vi "TURCK GUI TestPanel alle Module.vi"() -> ()   [LabVIEW 2017]
doc: "Example for reading and writing values for the TBEN-S2-2RFID-4DXP module from Turck"
uses:
  KH TURCK ETHERNETIP TDef Enum RFID Error.ctl
  KH TURCK ETHERNETIP TDefCluster TBEN-S2-2RFID-4DXP Status.ctl
  KH EthernetIPConfig 17.14/KH EthernetIPConfig TDef Config.ctl
  KH EthernetIPConfig 17.14/KH EthernetIPConfig TypeDefs ModuleTyp.ctl
  KH_DAQ 17.04/Turck/KH_DAQ_TURCK_TypeDefs_Cluster DI.ctl
  KH_DAQ 17.04/KH_DAQ_TypeDefs_Cluster AO.ctl
  KH_DAQ 17.04/KH_DAQ_TypeDefs_Messbereich.ctl
  KH_DAQ 17.04/KH_DAQ_TypeDefs_Bereich.ctl
  KH_DAQ 17.04/KH_DAQ_TypeDefs_Cluster AI.ctl
  KH TURCK ETHERNETIP TDef Enum IOL Data.ctl
  KH_DAQ 17.04/Turck/KH_DAQ_TURCK_TypeDefs_Cluster DO.ctl
  KH TURCK ETHERNETIP TDef Enum RFID Data RFID.ctl
  KH TURCK TypeDefs FGlob.ctl
  KH TURCK ETHERNETIP TDef Enum RFID User Command.ctl
  KH EthernetIP 17.19/KH_EthernetIP_Globals.vi
  KH TURCK ETHERNETIP RFID Global.vi
  KH TURCK ETHERNETIP RFID ST READ Global.vi
  KH TURCK ETHERNETIP Global.vi
panel:
  in  "Tab Control":T1(tab)
  in  "EIP_DO":T2={"Def"=[], "Signal Name"=["IOL1", "IOL3", "ARFID2", "ARFID3", "BRFID0", "BRFID1", "ADXP0", "ADXP2", "ADXP6", "ADXP7", "BDXP1", "BDXP2", "BDXP3", "BDXP7"], "Description"=[], "Chan"=[], "Inv"=[], "Nr"=[1, 1, 1, 1, 2, 2, 1, 1, 1, 1, 2, 2, 2, 2], "SensorType"=[enum."TBEN-S2-4IOL", enum."TBEN-S2-4IOL", enum."TBEN-S2-2RFID-4DXP", enum."TBEN-S2-2RFID-4DXP", enum."TBEN-S2-2RFID-4DXP", enum."TBEN-S2-2RFID-4DXP", enum."TBEN-S1-8DXP", enum."TBEN-S1-8DXP", enum."TBEN-S1-8DXP", enum."TBEN-S1-8DXP", enum."TBEN-S1-8DXP", enum."TBEN-S1-8DXP", enum."TBEN-S1-8DXP", enum."TBEN-S1-8DXP"]} {"Nr" max=63; "Chan" max=63}
  in  "EIP_DI":T4={"Signal Name"=["IOL0", "IOL2", "ARFID0", "ARFID1", "BRFID2", "BRFID3", "ADXP1", "ADXP3", "ADXP4", "ADXP5", "BDXP0", "BDXP4", "BDXP5", "BDXP6"], "Description"=[], "Chan"=[], "Inv"=[], "Nr"=[1, 1, 1, 1, 2, 2, 1, 1, 1, 1, 2, 2, 2, 2], "SensorType"=[enum."TBEN-S2-4IOL", enum."TBEN-S2-4IOL", enum."TBEN-S2-2RFID-4DXP", enum."TBEN-S2-2RFID-4DXP", enum."TBEN-S2-2RFID-4DXP", enum."TBEN-S2-2RFID-4DXP", enum."TBEN-S1-8DXP", enum."TBEN-S1-8DXP", enum."TBEN-S1-8DXP", enum."TBEN-S1-8DXP", enum."TBEN-S1-8DXP", enum."TBEN-S1-8DXP", enum."TBEN-S1-8DXP", enum."TBEN-S1-8DXP"]} {"Nr" max=63; "Chan" max=63}
  in  "EIP_AO":T5={"Signal Name"=["AO0 Modul1", "AO1 Modul1", "AO2 Modul1", "AO3 Modul1", "AO0 Modul2", "AO1 Modul2", "AO2 Modul2", "AO3 Modul2"], "Description"=[], "Phys Unit"=[], "Messbereich"=[enum."0V ... +10V", enum."0V ... +10V", enum."0V ... +10V", enum."0V ... +10V", enum."0V ... +10V", enum."0V ... +10V", enum."0V ... +10V", enum."0V ... +10V"], "Chan"=[], "Phys Min"=[0.0, 0.0, 0.0, 0.0, 0.0, 0.0, 0.0, 0.0], "Phys Max"=[10.0, 10.0, 10.0, 10.0, 10.0, 10.0, 10.0, 10.0], "Offset"=[], "Nr"=[], "SensorType 2"=[enum."TBEN-S2-4AO", enum."TBEN-S2-4AO", enum."TBEN-S2-4AO", enum."TBEN-S2-4AO", enum."TBEN-S2-4AO", enum."TBEN-S2-4AO", enum."TBEN-S2-4AO", enum."TBEN-S2-4AO"], "Bereich"=[enum."Standard", enum."Standard", enum."Standard", enum."Standard", enum."Standard", enum."Standard", enum."Standard", enum."Standard"], "Default"=[]} {"Offset" format="%.4f"; "Phys Max" format="%.4f"; "Phys Min" format="%.4f"}
  in  "EIP_AI":T8={"Signal Name"=["AI0 Modul 1", "AI1 Modul 1", "AI2 Modul 1", "AI3 Modul 1", "AI0 Modul 2", "AI1 Modul 2", "AI2 Modul 2", "AI3 Modul 2"], "Description"=[], "Phys Unit"=[], "Messbereich"=[enum."0 Ohm ... 4000 Ohm", enum."0 Ohm ... 4000 Ohm", enum."0 Ohm ... 4000 Ohm", enum."0 Ohm ... 4000 Ohm", enum."0 Ohm ... 4000 Ohm", enum."0 Ohm ... 4000 Ohm", enum."0 Ohm ... 4000 Ohm", enum."0 Ohm ... 4000 Ohm"], "Chan"=[], "Phys Min"=[0.0, 0.0, 0.0, 0.0, 0.0, 0.0, 0.0, 0.0], "Phys Max"=[10.0, 10.0, 10.0, 10.0, 10.0, 10.0, 10.0, 10.0], "Offset"=[], "Nr"=[], "SensorType 2"=[enum."TBEN-S2-4AI", enum."TBEN-S2-4AI", enum."TBEN-S2-4AI", enum."TBEN-S2-4AI", enum."TBEN-S2-4AI", enum."TBEN-S2-4AI", enum."TBEN-S2-4AI", enum."TBEN-S2-4AI"], "Bereich"=[enum."Standard", enum."Standard", enum."Standard", enum."Standard", enum."Standard", enum."Standard", enum."Standard", enum."Standard"]} {"Offset" format="%.4f"; "Phys Max" format="%.4f"; "Phys Min" format="%.4f"}
  in  "Config File":path=path "C:/LabView/Kirschenhofer/EIP/KH Turck EthernetIP 17.12/examples/ini alle Module 10.ini"
  in  "Parameter RFID Array":T9(array[cluster])=[{"NumberOfBytes0"=312, "SizeFragmentRead1"=128, "SizeFragmentRead0"=128, "SizeFragmentWrite0"=128, "SizeFragmentWrite1"=128, "NumberOfBytes1"=312}, {"NumberOfBytes0"=312, "SizeFragmentRead1"=128, "SizeFragmentRead0"=128, "SizeFragmentWrite0"=128, "SizeFragmentWrite1"=128, "NumberOfBytes1"=312}]
  in  "Config":T10[](array[typedef])=[{"Typ"=enum."TBEN-S2-4IOL", "Name"="1", "Nr."=1, "InputOutput"=[enum."Input", enum."Output", enum."Input", enum."Output"]}, {"Typ"=enum."TBEN-S2-4AO", "Name"="2", "Nr."=1, "InputOutput"=[enum."Output", enum."Output", enum."Output", enum."Output"]}, {"Typ"=enum."TBEN-S2-4AO", "Name"="", "Nr."=2, "InputOutput"=[enum."Output", enum."Output", enum."Output", enum."Output"]}, {"Typ"=enum."TBEN-S2-2RFID-4DXP", "Name"="", "Nr."=1, "InputOutput"=[enum."Input", enum."Input", enum."Output", enum."Output"]}, {"Typ"=enum."TBEN-S2-2RFID-4DXP", "Name"="", "Nr."=2, "InputOutput"=[enum."Output", enum."Output", enum."Input", enum."Input"]}, {"Typ"=enum."TBEN-S1-8DXP", "Name"="", "Nr."=1, "InputOutput"=[enum."Output", enum."Input", enum."Output", enum."Input", enum."Input", enum."Input", enum."Output", enum."Output"]}, {"Typ"=enum."TBEN-S1-8DXP", "Name"="", "Nr."=2, "InputOutput"=[enum."Input", enum."Output", enum."Output", enum."Output", enum."Input", enum."Input", enum."Input", enum."Output"]}, {"Typ"=enum."TBEN-S2-4AI", "Name"="", "Nr."=1, "InputOutput"=[enum."Input", enum."Input", enum."Input", enum."Input"]}, {"Typ"=enum."TBEN-S2-4AI", "Name"="", "Nr."=2, "InputOutput"=[enum."Input", enum."Input", enum."Input", enum."Input"]}]
  in  "Write Kanal 0 Modul 1":u8[](array[numeric])
  in  "Write Kanal 1 Modul 1":u8[](array[numeric])
  in  "Write Kanal 0 Modul 2":u8[](array[numeric])
  in  "Write Kanal 1 Modul 2":u8[](array[numeric])
  out "Kanal 0 Modul 1":u8[](array[numeric])
  out "Kanal 0 Modul 2":u8[](array[numeric])
  out "Kanal 1 Modul 2":u8[](array[numeric])
  out "Kanal 1 Modul 1":u8[](array[numeric])
  out "UID Kanal 1 Modul 1":u8[](array[numeric])
  out "UID Kanal 1 Modul 2":u8[](array[numeric])
  out "UID Kanal 0 Modul2":u8[](array[numeric])
  out "UID Kanal 0 Modul 1":u8[](array[numeric])
  out "Error0 Modul 1":T11=33282
  out "Error1 Modul 1":T11=33282
  out "Error1 Modul 2":T11=33282
  out "Error0 Modul 2":T11=33282
  in  "Read":bool[](array[boolean])
  in  "Write":bool[](array[boolean])
  in  "Inventory":bool[](array[boolean])
  in  "Reset message":bool caption="Button"
  in  "TagNr":enum16{"Tag 0", "Tag 1"}(ring)
  out "Status Array":T12[](array[typedef])=[{"Error writing 1"=FALSE, "ReadingFinished 1"=FALSE, "WritingFinished 1"=FALSE, "Error writing 0"=FALSE, "ReadingFinished 0"=FALSE, "WritingFinished 0"=FALSE, "Timeout 1"=FALSE, "State0"="Idle", "State1"="Start", "Timeout 0"=FALSE, "Successfull Writing 1"=FALSE, "Successfull Writing 0"=FALSE}, {"Error writing 1"=FALSE, "ReadingFinished 1"=FALSE, "WritingFinished 1"=FALSE, "Error writing 0"=FALSE, "ReadingFinished 0"=FALSE, "WritingFinished 0"=FALSE, "Timeout 1"=TRUE, "State0"="", "State1"="", "Timeout 0"=FALSE, "Successfull Writing 1"=FALSE, "Successfull Writing 0"=FALSE}]
  out "RFID 0 Read SM":T13[](array[typedef])
  out "RFID 1 Read SM":T13[](array[typedef])
  out "DXP2":bool[](array[boolean])
  in  "DXP Status":string[](array[string])=["Channel 0 - Overcurrent", "Channel 1 - Overcurrent", "Channel 2 - Overcurrent", "Channel 3 - Overcurrent", "Channel 4 - Overcurrent", "Channel 5 - Overcurrent", "Channel 6 - Overcurrent", "Channel 7 - Overcurrent", "Overcurrent VAUX1 Ch0-3", "Overcurrent VAUX2 Ch4-7", "Channel 0 - Latch input", "Channel 1 - Latch input", "Channel 2 - Latch input", "Channel 3 - Latch input", "Channel 4 - Latch input", "Channel 5 - Latch input", "Channel 6 - Latch input", "Channel 7 - Latch input", "Module Diagnostics Available", "INFO: ARGEE Project Running", "Undervoltage V2", "Undervoltage V1", "Force Mode Enabled"]
  out "DXP1":bool[](array[boolean])
  out "AI2":bool[](array[boolean])
  in  "AI Status":string[](array[string])=["upper limit CH0", "upper limit CH1", "upper limit CH2", "upper limit CH3", "Overflow CH0", "Overflow CH1", "Overflow CH2", "Overflow CH3", "Underflow CH0", "Underflow CH1", "Underflow CH2", "Underflow CH3", "CJC Wire Break CH0", "CJC Wire Break CH1", "CJC Wire Break CH2", "CJC Wire Break CH3", "Overcurrent (RTD) CH0", "Overcurrent (RTD) CH1", "Overcurrent (RTD) CH2", "Overcurrent (RTD) CH3", "Wire break CH0", "Wire break CH1", "Wire break CH2", "Wire break CH3", "Overcurrent supply VAUX1 CH0", "Overcurrent supply VAUX1 CH1", "Overcurrent supply VAUX1 CH2", "Overcurrent supply VAUX1 CH3", "Lower limit value underrun CH0", "Lower limit value underrun CH1", "Lower limit value underrun CH2", "Lower limit value underrun CH3", "Module Diagnostics Available", "INFO: ARGEE Project Running", "Undervoltage Field Supply V2", "Undervoltage Field Supply V1", "Internal Error", "Force Mode Enabled"]
  out "AI":sgl[](array[numeric]) format="%.6f"
  out "AI1":bool[](array[boolean])
  in  "AO Status":string[](array[string])=["Modul 1 Overload Ch0", "Modul 1 Overload Ch1", "Modul 1 Overload Ch2", "Modul 1 Overload Ch3", "Modul 1 Wirebreak Ch0", "Modul 1 Wirebreak Ch1", "Modul 1 Wirebreak Ch2", "Modul 1 Wirebreak Ch3", "Modul 1 Module Diagnostics Available", "Modul 1 INFO: ARGEE Project Running", "Modul 1 Undervoltage V2", "Modul 1 Undervoltage V1", "Modul 1 Internal Error", "Modul 1 Force Mode Enabled", "Modul 2 Overload Ch0", "Modul 2 Overload Ch1", "Modul 2 Overload Ch2", "Modul 2 Overload Ch3", "Modul 2 Wirebreak Ch0", "Modul 2 Wirebreak Ch1", "Modul 2 Wirebreak Ch2", "Modul 2 Wirebreak Ch3", "Modul 2 Module Diagnostics Available", "Modul 2 INFO: ARGEE Project Running", "Modul 2 Undervoltage V2", "Modul 2 Undervoltage V1", "Modul 2 Internal Error", "Modul 2 Force Mode Enabled"]
  out "AO Status":bool[](array[boolean])
  in  "AO Values":sgl[](array[numeric])=[0.0, 0.0, 0.0, 0.0, 0.0, 0.0, 0.0, 0.0] format="%.6f"
  in  "Output_IOL":T14={"IOL Port 1"=[0, 0], "IOL Port 2"=[0, 0], "IOL Port 3"=[0, 0], "IOL Port 4"=[0, 0]}
  out "IOL":T15
  out "DI":bool[](array[boolean])
  in  "DI":string[](array[string])=["IOL0", "IOL2", "ARFID0", "ARFID1", "BRFID2", "BRFID3", "ADXP1", "ADXP3", "ADXP4", "ADXP5", "BDXP0", "BDXP4", "BDXP5", "BDXP6"]
  in  "Reset 0":bool
  in  "Reset 1":bool
  in  "Reset 2":bool
  in  "Reset 3":bool
  in  "Reset 4":bool
  in  "Reset 5":bool
  in  "Reset 6":bool
  in  "Reset 7":bool
  in  "DO":bool[](array[boolean])=[FALSE, FALSE, FALSE, FALSE, FALSE, FALSE, FALSE, FALSE, FALSE, FALSE, FALSE, FALSE, FALSE, FALSE]
  out "DO in":bool[](array[boolean])
  in  "Signal Name":string[](array[string])=["IOL1", "IOL3", "ARFID2", "ARFID3", "BRFID0", "BRFID1", "ADXP0", "ADXP2", "ADXP6", "ADXP7", "BDXP1", "BDXP2", "BDXP3", "BDXP7"]
  out "error out":errorcluster
  in  "Exit":bool
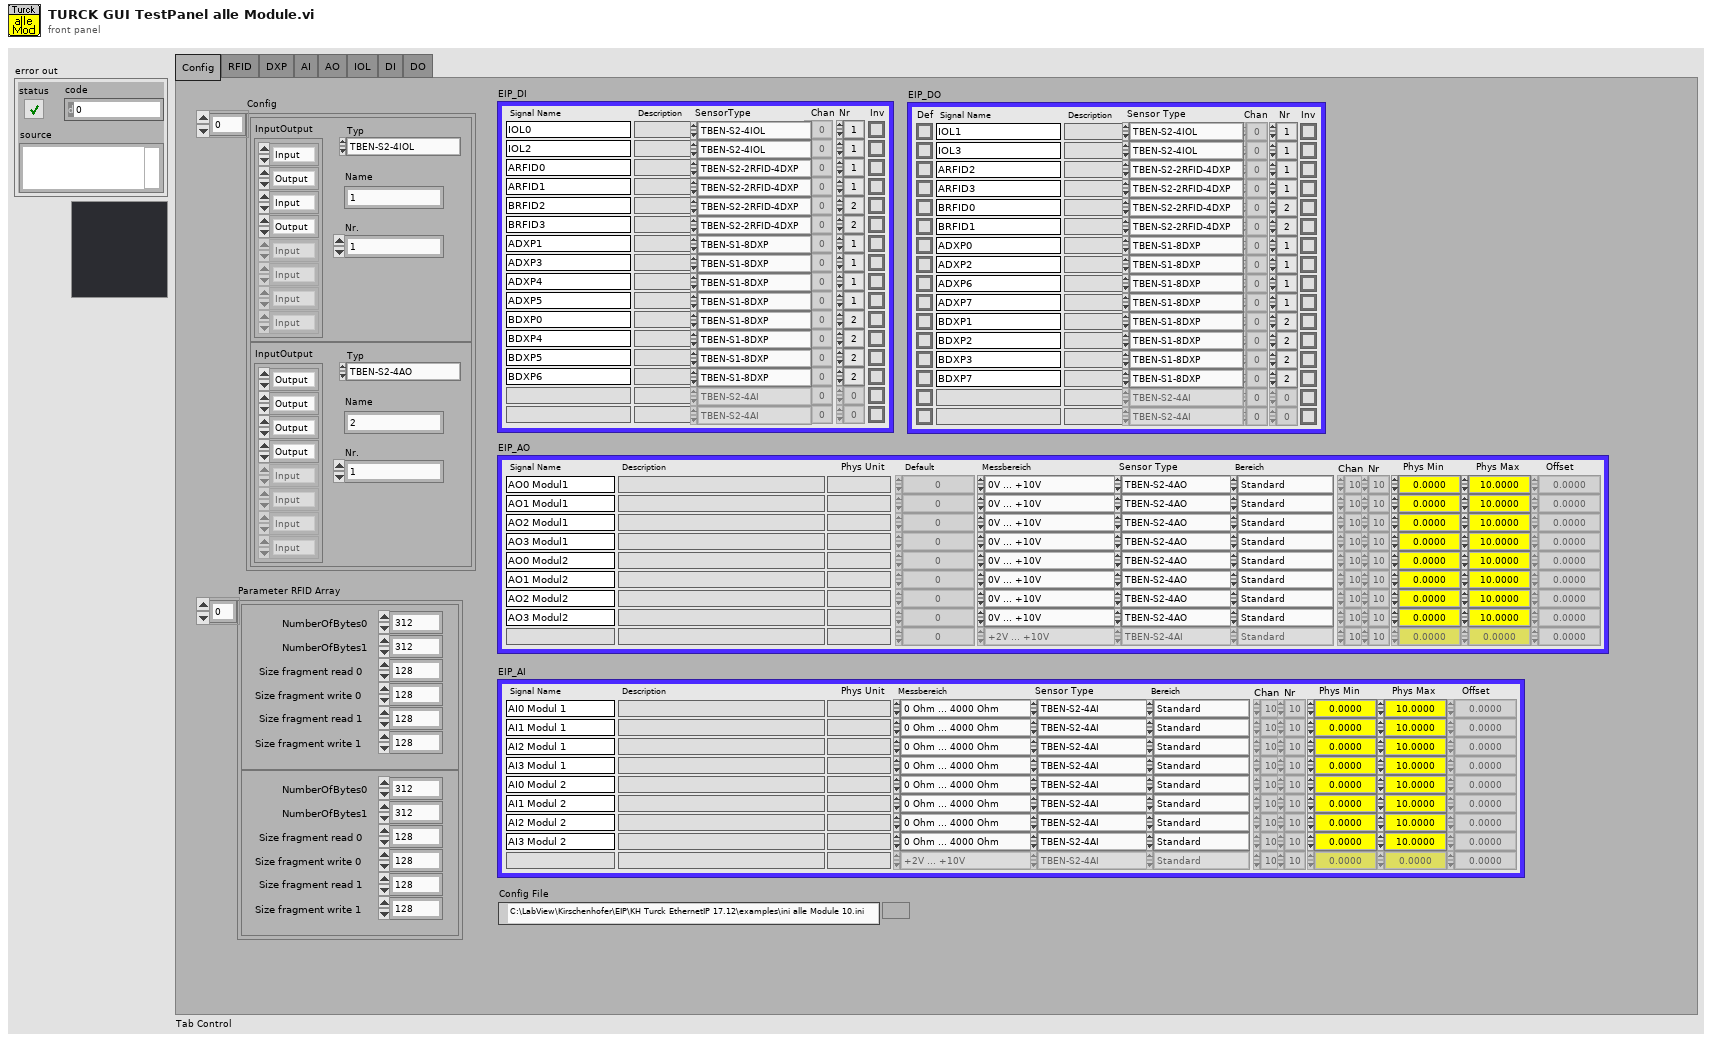
[diagram p1: front panel]
types:
  T1 = enum32{"Config", "RFID", "DXP", "AI", "AO", "IOL", "DI", "DO"}
  T2 = typedef "KH_DAQ_TURCK_TypeDefs_Cluster DO.ctl" = cluster{"Def":bool[], "Signal Name":string[], "Description":string[], "Chan":u16[], "Inv":bool[], "Nr":u16[], "SensorType":T3[]}
  T3 = typedef "KH EthernetIPConfig TypeDefs ModuleTyp.ctl" = enum16{"TBEN-S2-4AI", "TBEN-S1-8DXP", "TBEN-S2-2RFID-4DXP", "TBEN-S2-4AO", "TBEN-S2-4IOL"}
  T4 = typedef "KH_DAQ_TURCK_TypeDefs_Cluster DI.ctl" = cluster{"Signal Name":string[], "Description":string[], "Chan":u16[], "Inv":bool[], "Nr":u16[], "SensorType":T3[]}
  T5 = typedef "KH_DAQ_TypeDefs_Cluster AO.ctl" = cluster{"Signal Name":string[], "Description":string[], "Phys Unit":string[], "Messbereich":T6[], "Chan":u16[], "Phys Min":sgl[], "Phys Max":sgl[], "Offset":sgl[], "Nr":u16[], "SensorType 2":T3[], "Bereich":T7[], "Default":sgl[]}
  T6 = typedef "KH_DAQ_TypeDefs_Messbereich.ctl" = enum16{"-10V ... +10V", "0V ... +10V", "+2V ... +10V", "0V ... +5V", "+1V ... +5V", "-1V ... +1V", "-500mV ... +500mV", "-100mV ... +100mV", "-50mV ... +50mV", "0mA ... +20mA", "+4mA ... +20mA", "-20mA ... +20mA", "0 Ohm ... 100 Ohm", "0 Ohm ... 400 Ohm", "0 Ohm ... 2000 Ohm", "0 Ohm ... 4000 Ohm", "-200°C ... 150°C PT100", "-200°C ... 150°C PT200", "-200°C ... 150°C PT500", "-200°C ... 150°C PT1000", "-60°C ... 150°C Ni100", "-60°C ... 150°C Ni1000", "-200°C ... 850°C PT100", "-200°C ... 850°C PT200", "-200°C ... 850°C PT500", "-200°C ... 850°C PT1000", "-50°C ... 250°C Ni100", "-50°C ... 250° Ni 1000"}
  T7 = typedef "KH_DAQ_TypeDefs_Bereich.ctl" = enum16{"Standard", "extended Range", "NE43", ""}
  T8 = typedef "KH_DAQ_TypeDefs_Cluster AI.ctl" = cluster{"Signal Name":string[], "Description":string[], "Phys Unit":string[], "Messbereich":T6[], "Chan":u16[], "Phys Min":sgl[], "Phys Max":sgl[], "Offset":sgl[], "Nr":u16[], "SensorType 2":T3[], "Bereich":T7[]}
  T9 = cluster{"NumberOfBytes0":i32, "SizeFragmentRead1":i32, "SizeFragmentRead0":i32, "SizeFragmentWrite0":i32, "SizeFragmentWrite1":i32, "NumberOfBytes1":i32}[]
  T10 = typedef "KH EthernetIPConfig TDef Config.ctl" = cluster{"Typ":T3, "Name":string, "Nr.":i32, "InputOutput":enum16{"Input", "Output"}[]}
  T11 = typedef "KH TURCK ETHERNETIP TDef Enum RFID Error.ctl" = u16
  T12 = typedef "KH TURCK ETHERNETIP TDefCluster TBEN-S2-2RFID-4DXP Status.ctl" = cluster{"Error writing 1":bool, "ReadingFinished 1":bool, "WritingFinished 1":bool, "Error writing 0":bool, "ReadingFinished 0":bool, "WritingFinished 0":bool, "Timeout 1":bool, "State0":string, "State1":string, "Timeout 0":bool, "Successfull Writing 1":bool, "Successfull Writing 0":bool}
  T13 = typedef "KH TURCK ETHERNETIP TDef Enum RFID Data RFID.ctl" = cluster{"ResponseCode":u16, "LoopCounter":u8, "Length":u16, "WriteFragmentNo":u8, "ReadFragmentNo":u8, "Data":u8[], "TagPresent":bool, "Error":bool, "BusyFinished":bool, "Channel":u16}
  T14 = cluster{"IOL Port 1":u16[], "IOL Port 2":u16[], "IOL Port 3":u16[], "IOL Port 4":u16[]}
  T15 = typedef "KH TURCK ETHERNETIP TDef Enum IOL Data.ctl" = cluster{"Data_Port1":u16[], "Data_Port3":u16[], "Data_Port5":u16[], "Data_Port7":u16[], "Status":cluster{"Undervoltage Field Supply V2":bool, "Overvoltage Field Supply V1":bool, "Undervoltage Field Supply V1":bool, "Internal Error":bool, "Module Diagnostics Available":bool, "Station Configuration Changed":bool, "Overcurrent Isys":bool, "Overvoltage Field Supply V2":bool, "Force Mode Enabled":bool}, "Diagnostics":cluster{"Channel 2 - Output signal overcurrent":bool, "Channel 4 - Output signal overcurrent":bool, "Channel 6 - Output signal overcurrent":bool, "Channel 8 - Output signal overcurrent":bool, "Channel 1 - Wrong or missing device":bool, "Channel 3 - Wrong or missing device":bool, "Channel 5 - Wrong or missing device":bool, "Channel 7 - Wrong or missing device":bool, "Channel 1 - Data storage error":bool, "Channel 3 - Data storage error":bool, "Channel 5 - Data storage error":bool, "Channel 7 - Data storage error":bool, "Channel 1 - Process input data invalid":bool, "Channel 3 - Process input data invalid":bool, "Channel 5 - Process input data invalid":bool, "Channel 7 - Process input data invalid":bool, "Channel 1 - Hardware error":bool, "Channel 3 - Hardware error":bool, "Channel 5 - Hardware error":bool, "Channel 7 - Hardware error":bool, "Channel 1 - Maintenance events":bool, "Channel 3 - Maintenance events":bool, "Channel 5 - Maintenance events":bool, "Channel 7 - Maintenance events":bool, "Channel 1 - Out of spec. error":bool, "Channel 3 - Out of spec. error":bool, "Channel 5 - Out of spec. error":bool, "Channel 7 - Out of spec. error":bool, "Channel 1 - Parameterization error":bool, "Channel 3 - Parameterization error":bool, "Channel 5 - Parameterization error":bool, "Channel 1 - Overtemperature":bool, "Channel 3 - Overtemperature":bool, "Channel 5 - Overtemperature":bool, "Channel 7 - Overtemperature":bool, "Channel 1 - Lower limit value underrun":bool, "Channel 3 - Lower limit value underrun":bool, "Channel 5 - Lower limit value underrun":bool, "Channel 7 - Lower limit value underrun":bool, "Channel 1 - Upper limit value exceeded":bool, "Channel 3 - Upper limit value exceeded":bool, "Channel 5 - Upper limit value exceeded":bool, "Channel 7 - Upper limit value exceeded":bool, "Channel 1 - Undervoltage":bool, "Channel 3 - Undervoltage":bool, "Channel 5 - Undervoltage":bool, "Channel 7 - Undervoltage":bool, "Channel 1 - Overvoltage":bool, "Channel 3 - Overvoltage":bool, "Channel 5 - Overvoltage":bool, "Channel 7 - Overvoltage":bool, "Channel 1 - Overload":bool, "Channel 3 - Overload":bool, "Channel 5 - Overload":bool, "Channel 7 - Overload":bool, "Channel 1 - Common error":bool, "Channel 3 - Common error":bool, "Channel 5 - Common error":bool, "Channel 7 - Common error":bool, "Channel 1 - Port parameterization error":bool, "Channel 3 - Port parameterization error":bool, "Channel 5 - Port parameterization error":bool, "Channel 7 - Parameterization error":bool, "Channel 7 - Port parameterization error":bool}, "Events":cluster{"Event":u8[], "Qualifier":u8[], " Event code":u16[]}, "DXP":cluster{"DI Input value 2":bool, "DI Input value 4":bool, "DI Input value 6":bool, "DI Input value 8":bool, "DI Input 1":bool, "DI Input 3":bool, "DI Input 5":bool, "DI Input 7":bool, "Input values valid 1":bool, "Input values valid 3":bool, "Input values valid 5":bool, "Input values valid 7":bool}}
  T16 = typedef "KH TURCK ETHERNETIP TDef Enum RFID User Command.ctl" = enum16{"read", "write", "idle", "inventory"}
  T17 = typedef "KH TURCK TypeDefs FGlob.ctl" = enum16{"Put one", "Put all", "Recall one", "Recall all"}
  T18 = typedef "KH TURCK ETHERNETIP TDefCluster TURCK RFID.ctl" = cluster{"NumberOfBytes":i32, "State":string, "Counter":i32, "ReadData":u8[], "AnzahlFragmente":i32, "WritingFinished":bool, "ReadingFinished":bool, "UID":u8[], "ActCommand":T19, "SizeFragmentRead":i32, "LengthUID":u16, "WriteDataInclUID":u8[], "Timeout":bool, "SizeFragmentWrite":i32}
  T19 = typedef "KH TURCK ETHERNETIP TDef Enum RFID Act Command.ctl" = enum16{"read", "write", "idle", "Inventory", ""}
  T20 = typedef "KH TURCK ETHERNETIP TDefCluster TBEN-S2-2RFID-4DXP Input Values.ctl" = cluster{"Station Status Word (Input Data Mapping)":cluster{"Module diagnostics avaliable":bool, "INFO: ARGEE Project Running":bool, "Undervoltage V2":bool, "Undervoltage V1":bool, "Internal Error":bool, "I/O-ASSISTANT Force Mode active":bool}, "RFID control/status 0 (Input Data Mapping)":cluster{"Tag present at r/w head":bool[], "response code":u16, "loop counter":u8, "Length":u16, "Error code":u16, "Tag counter":u16, "Data (Bytes) available":u16, "Read fragment No.":u8, "Write fragment No.":u8, "Tag present at r/w head bit":bool, "HF r/w head switched on":bool, "Continuous mode active":bool, "Antenna detuned at HF read/write head":bool, "Parameter not supported by read/write head":bool, "Error reported by read/write head":bool, "Not connected to read/write head":bool}, "RFID read data 0 (Input Data Mapping)":u8[], "RFID control/status 1 (Input Data Mapping)":cluster{"response code":u16, "Loop counter":u8, "Length":u16, "Error code":u16, "Tag counter":u16, "Data (Bytes) available":u16, "Read fragment No.":u8, "Write fragment No.":u8, "Tag present at r/w head bit":bool, "HF r/w head switched on":bool, "Continuous mode active":bool, "Antenna detuned at HF read/write head":bool, "Parameter not supported by read/write head":bool, "Error reported by read/write head":bool, "Not connected to read/write head":bool, "Tag present at r/w head":bool[]}, "RFID read data 1 (Input Data Mapping)":u8[], "RFID diagnostics (Input Data Mapping)":cluster{"Overcurrent supply VAUX1 (a)":bool, "Parameterization error (a)":bool, "Configuration via DTM active (a)":bool, "Buffer full (a)":bool, "Antenna detuned at HF read/write head (a)":bool[], "Parameter not supported by read/write head (a)":bool[], "Error reported by read/write head (a)":bool[], "Not connected to read/write head (a)":bool[], "Overcurrent supply VAUX1 (b)":bool, "Parameterization error (b)":bool, "Configuration via DTM active (b)":bool, "Buffer full (b)":bool, "Antenna detuned at HF read/write head (b)":bool[], "Parameter not supported by read/write head (b)":bool[], "Error reported by read/write head (b)":bool[], "Not connected to read/write head (b)":bool[]}, "DXP diagnostics (Input Data Mapping)":cluster{"Overcurrent VAUX2 Ch4/5":bool, "Overcurrent VAUX2 Ch6/7":bool, "Channel 4 - Output overcurrent":bool, "Channel 5 - Output overcurrent":bool, "Channel 6 - Output overcurrent":bool, "Channel 7 - Output overcurrent":bool}, "DXP (Input Data Mapping)":cluster{"Channel 4 - Input value":bool, "Channel 5 - Input value":bool, "Channel 6 - Input value":bool, "Channel 7 - Input value":bool}}
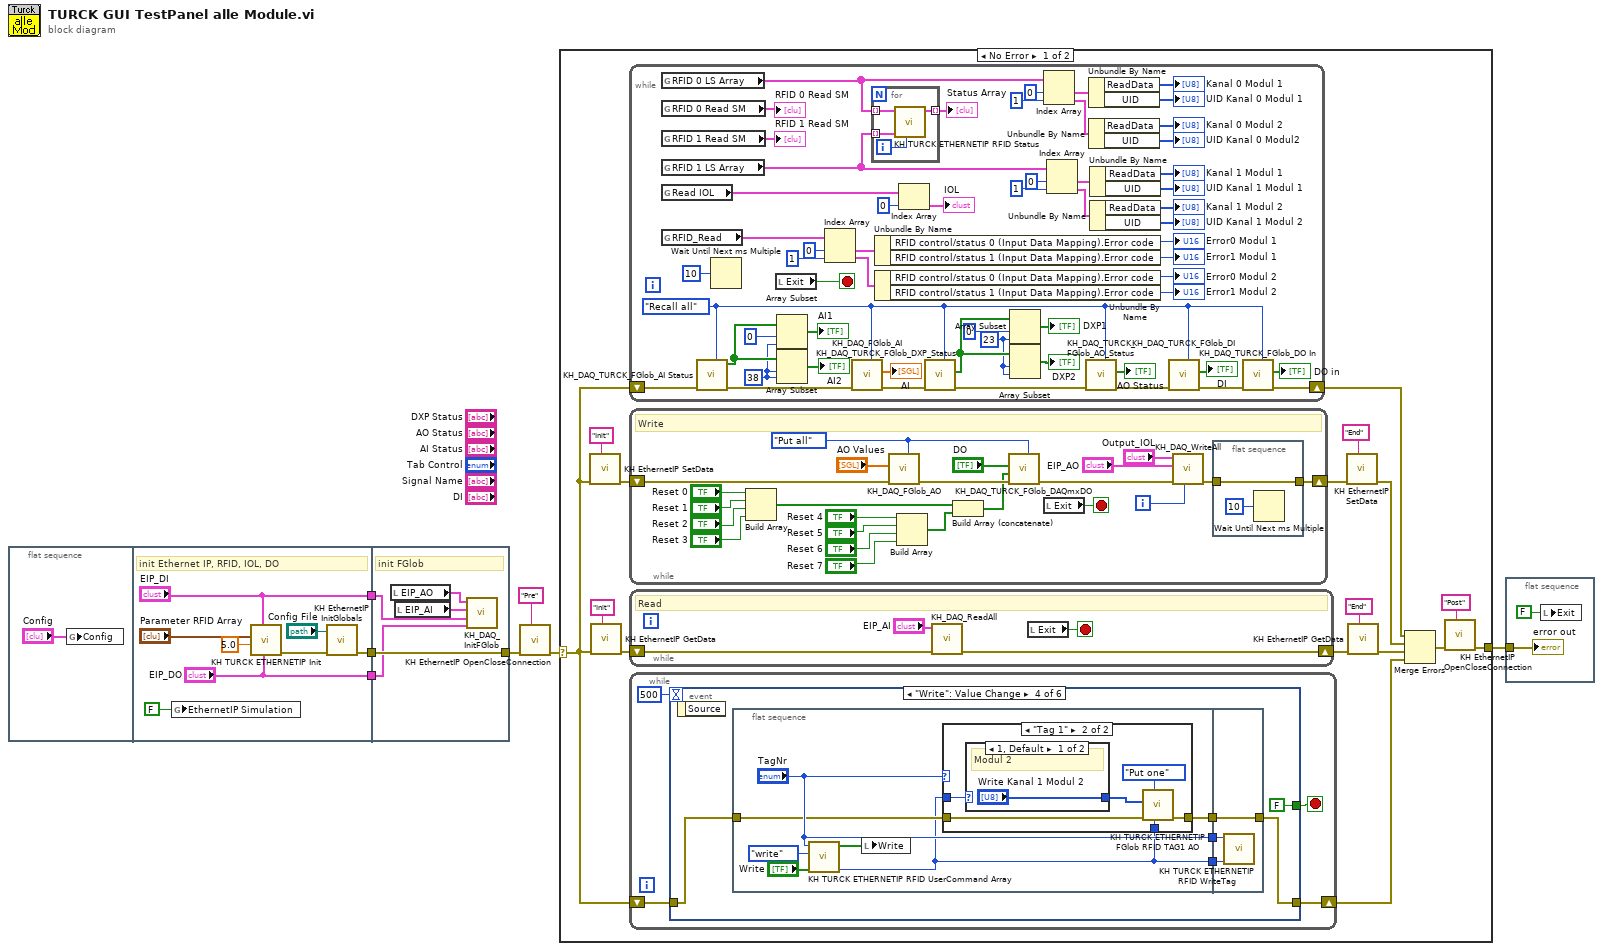
[diagram p0: block diagram]
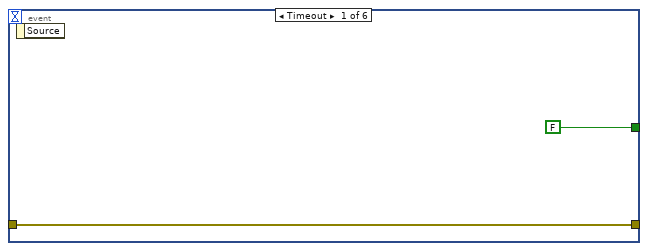
[diagram p2: hidden frame]
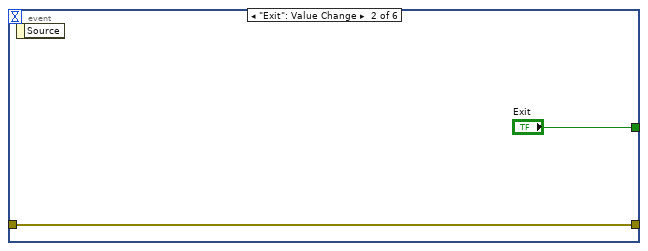
[diagram p3: hidden frame]
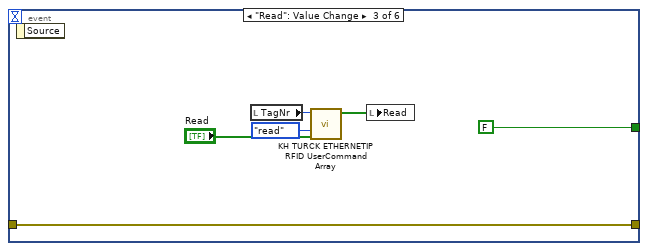
[diagram p4: hidden frame]
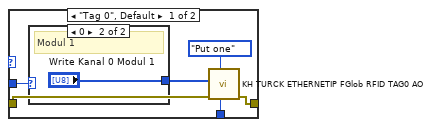
[diagram p5: hidden frame]
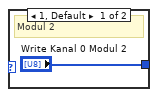
[diagram p6: hidden frame]
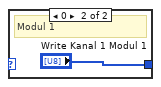
[diagram p7: hidden frame]
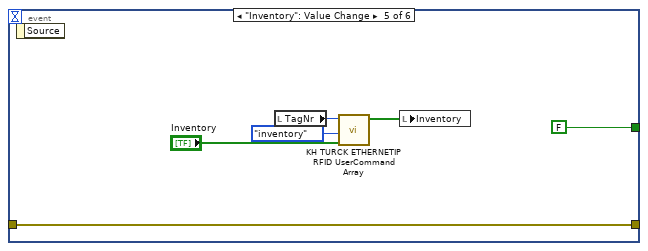
[diagram p8: hidden frame]
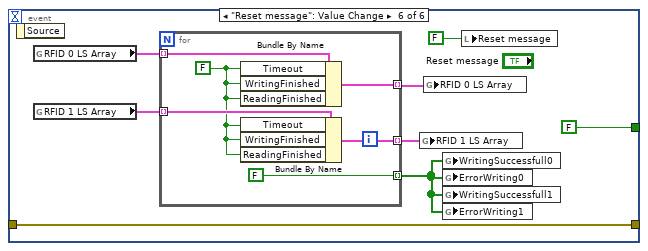
[diagram p9: hidden frame]
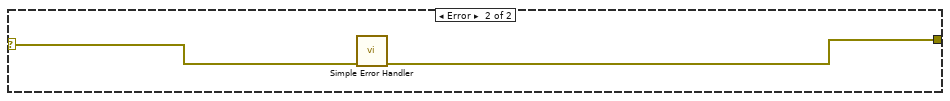
[diagram p10: hidden frame]
diagram:
  n1 = flat-sequence {
    tunnel: [w16] -> w3
    tunnel: ["EIP_DI"] -> w2
    tunnel: ["EIP_DO"] -> w1
    tunnel: [w19] -> w5
    tunnel: w3 -> [w19]
    tunnel: w2 -> [w18]
    tunnel: w1 -> [w17]
    frame #0 {
      n2 = global write "KH_EthernetIP_Globals.vi" "Config"("Config") -> ()
    }
    frame #1 {
      # "init Ethernet IP, RFID, IOL, DO"
      n3 = global write "KH_EthernetIP_Globals.vi" "EthernetIP Simulation"(FALSE ("EthernetIP Simulation")) -> ()
      n4 = call "KH TURCK ETHERNETIP Init.vi"("EIP_DO"="EIP_DO", "EIP_DI"="EIP_DI", "TimeoutRFID"=5.0 ("Timeout"), "Parameter RFID Array"="Parameter RFID Array") -> ("err out"=w12:errorcluster)  [unwired: 7 in]
      n5 = call "KH EthernetIP InitGlobals.vi"("err in"=w12, "Config File"="Config File") -> ("err out"=w16:errorcluster)  [unwired: 9 in]
    }
    frame #2 {
      # "init FGlob"
      n6 = local read "EIP_AO"() -> (w20:T5)
      n7 = local read "EIP_AI"() -> (w21:T8)
      n8 = call "KH_DAQ_InitFGlob.vi"("EIP_DO"=w17, "EIP_DI"=w18, "EIP_AI"=w21, "EIP_AO"=w20) -> ()  [unwired: 8 in]
    }
  }
  n9 = call "KH EthernetIP OpenCloseConnection.vi"("Function"="Pre", "error in"=w5) -> ("error out"=w6:errorcluster)  [unwired: 9 in]
  n10 = case shown="No Error" w6 {
    selector: w6 -> [w22 w195]
    tunnel: [w25 w194] -> w4
    frame No Error {
      n11 = call "KH EthernetIP SetData.vi"("Function"="Init", "error in"=w22) -> ("error out"=w24:errorcluster)  [unwired: 7 in, 2 out]
      n12 = call "KH EthernetIP GetData.vi"("Function"="Init", "error in"=w22) -> ("error out"=w37:errorcluster)  [unwired: 8 in, 1 out]
      n13 = while {
        shift-right: [w89] -> w23
        shift-left: w22 -> [w51]
        stop <- w88 stop-if-true
        w40 = 23 ("length")
        w57 = 38 ("index")
        w87 = KH_TURCK_TypeDefs_FGlob."Recall all" ("Function (Recall One)")
        n14 = global read "KH TURCK ETHERNETIP RFID Global.vi" "RFID 0 LS Array"() -> (w70:T18[])
        n15 = global read "KH TURCK ETHERNETIP RFID ST READ Global.vi" "RFID 0 Read SM"() -> (→"RFID 0 Read SM":T13[])
        n16 = global read "KH TURCK ETHERNETIP RFID ST READ Global.vi" "RFID 1 Read SM"() -> (→"RFID 1 Read SM":T13[])
        n17 = global read "KH TURCK ETHERNETIP RFID Global.vi" "RFID 1 LS Array"() -> (w76:T18[])
        n18 = global read "KH TURCK ETHERNETIP Global.vi" "Read IOL"() -> (w38:T15[])
        n19 = global read "KH TURCK ETHERNETIP Global.vi" "RFID_Read"() -> (w39:T20[])
        n20 = call "KH_DAQ_TURCK_FGlob_AI Status.vi"("Function (Recall One)"=w87, "err in"=w51) -> ("err out"=w94:errorcluster, "StatusOut"=w59:bool[])  [unwired: 7 in, 1 out]
        n21 = Wait Until Next ms Multiple(millisecond multiple=u32 10) -> ()  [unwired: 1 out]
        n22 = local read "Exit"() -> (w88:bool)
        n23 = Array Subset(array=w59, index=0, length=w57) -> (→"AI1":bool[])
        n24 = Array Subset(array=w59, index=w57, length=w57) -> (→"AI2":bool[])
        n25 = Index Array(array=w39, index #1=0 ("index"), index #2=1 ("index")) -> (element #1=w80:T20, element #2=w45:T20)
        n26 = call "KH_DAQ_FGlob_AI.vi"("Function (Recall One)"=w87, "err in"=w94) -> ("err out"=w93:errorcluster, "AI Values OUT"=→"AI":sgl[])  [unwired: 6 in, 2 out]
        n27 = for {
          tunnel: w70 -> [w98] mode=indexing
          tunnel: w76 -> [w97] mode=indexing
          tunnel: [w96] -> w65 mode=indexing
          i -> [w95]
          n28 = call "KH TURCK ETHERNETIP RFID Status.vi"("Nr.Module"=w95, "RFID 1"=w97, "RFID 0"=w98) -> ("StatusOUT"=w96:T12)  [unwired: 8 in]
        }
        "Status Array" <- w65
        n29 = Unbundle By Name(w80) -> ("RFID control/status 0 (Input Data Mapping).Error code"=→"Error0 Modul 1":u16, "RFID control/status 1 (Input Data Mapping).Error code"=→"Error1 Modul 1":u16)
        n30 = Unbundle By Name(w45) -> ("RFID control/status 0 (Input Data Mapping).Error code"=→"Error0 Modul 2":u16, "RFID control/status 1 (Input Data Mapping).Error code"=→"Error1 Modul 2":u16)
        n31 = Index Array(array=w38, index=0) -> (element=→"IOL":T15)
        n32 = call "KH_DAQ_TURCK_FGlob_DXP_Status.vi"("Function (Recall One)"=w87, "err in"=w93) -> ("err out"=w92:errorcluster, "DXP Status OUT"=w44:bool[])  [unwired: 8 in]
        n33 = Array Subset(array=w44, index=0, length=w40) -> (→"DXP1":bool[])
        n34 = Array Subset(array=w44, index=w40, length=w40) -> (→"DXP2":bool[])
        n35 = Index Array(array=w70, index #1=0 ("index"), index #2=1 ("index")) -> (element #1=w66:T18, element #2=w50:T18)
        n36 = Index Array(array=w76, index #1=0 ("index"), index #2=1 ("index")) -> (element #1=w74:T18, element #2=w47:T18)
        n37 = call "KH_DAQ_TURCK_FGlob_AO_Status.vi"("Function (Recall One)"=w87, "err in"=w92) -> ("err out"=w91:errorcluster, "AO Status OUT"=→"AO Status":bool[])  [unwired: 8 in]
        n38 = Unbundle By Name(w66) -> ("ReadData"=→"Kanal 0 Modul 1":u8[], "UID"=→"UID Kanal 0 Modul 1":u8[])
        n39 = Unbundle By Name(w50) -> ("ReadData"=→"Kanal 0 Modul 2":u8[], "UID"=→"UID Kanal 0 Modul2":u8[])
        n40 = Unbundle By Name(w74) -> ("ReadData"=→"Kanal 1 Modul 1":u8[], "UID"=→"UID Kanal 1 Modul 1":u8[])
        n41 = Unbundle By Name(w47) -> ("ReadData"=→"Kanal 1 Modul 2":u8[], "UID"=→"UID Kanal 1 Modul 2":u8[])
        n42 = call "KH_DAQ_TURCK_FGlob_DI.vi"("Function (Recall One)"=w87, "err in"=w91) -> ("err out"=w90:errorcluster, "DI Values OUT"=→"DI":bool[])  [unwired: 7 in, 1 out]
        n43 = call "KH_DAQ_TURCK_FGlob_DO In.vi"("Function (Recall One)"=w87, "err in"=w90) -> ("err out"=w89:errorcluster, "DO in Values OUT"=→"DO in":bool[])  [unwired: 7 in, 1 out]
      }
      n44 = while {
        shift-right: [w118] -> w28
        shift-left: w24 -> [w112]
        i -> [w117]
        stop <- w121 stop-if-true
        w113 = KH_TURCK_TypeDefs_FGlob."Put all" ("Function (Recall One)")
        # "Write"
        n45 = Build Array("Reset 0", "Reset 1", "Reset 2", "Reset 3") -> (w101:bool[])
        n46 = call "KH_DAQ_FGlob_AO.vi"("Function (Recall One)"=w113, "err in"=w112, "AO Values IN"="AO Values") -> ("err out"=w106:errorcluster)  [unwired: 6 in, 2 out]
        n47 = Build Array("Reset 4", "Reset 5", "Reset 6", "Reset 7") -> (w100:bool[])
        n48 = Build Array (concatenate)(w101, w100) -> (w99:bool[])
        n49 = call "KH_DAQ_TURCK_FGlob_DAQmxDO.vi"("Function (Recall One)"=w113, "err in"=w106, "DXP Reset IN"=w99, "DXP Values IN"="DO") -> ("err out"=w111:errorcluster)  [unwired: 4 in, 3 out]
        n50 = local read "Exit"() -> (w121:bool)
        n51 = call "KH_DAQ_WriteAll.vi"("Numeric"=w117, "err in"=w111, "EIP_AO"="EIP_AO", "Output_IOL"="Output_IOL") -> ("err out"=w119:errorcluster)  [unwired: 7 in]
        n52 = flat-sequence {
          tunnel: w119 -> [w122]
          tunnel: [w122] -> w118
          frame #0 {
            n53 = Wait Until Next ms Multiple(millisecond multiple=u32 10) -> ()  [unwired: 1 out]
          }
        }
      }
      n54 = while {
        shift-right: [w124] -> w35
        shift-left: w37 -> [w126]
        stop <- w127 stop-if-true
        # "Read"
        n55 = call "KH_DAQ_ReadAll.vi"("err in"=w126, "EIP_AI"="EIP_AI") -> ("err out"=w124:errorcluster)  [unwired: 9 in]
        n56 = local read "Exit"() -> (w127:bool)
      }
      n57 = while {
        shift-right: [w128] -> w26
        shift-left: w22 -> [w130]
        stop <- w131 stop-if-true
        n58 = event shown="[3] \"Write\": Value Change" {
          selector: _ -> [_ _ _ _ _ _]
          dyn-events: _ -> [_ _ _ _ _ _]
          timeout: 500 -> [_ _ _ _ _ _]
          tunnel: [FALSE ("Exit") "Exit" FALSE ("Exit") FALSE ("Exit") FALSE ("Exit") FALSE ("Exit")] -> w131
          tunnel: w130 -> [w132 w134 w140 w146 w178 w186]
          tunnel: [w132 w134 w140 w145 w178 w186] -> w128
          event Timeout {
            n59 = event-data() -> ()  [unwired: 1 in, 1 out]
          }
          event "Exit": Value Change {
            n60 = event-data() -> ()  [unwired: 1 in, 1 out]
          }
          event "Read": Value Change {
            n61 = event-data() -> ()  [unwired: 1 in, 1 out]
            n62 = local read "TagNr"() -> (w139:enum16{"Tag 0", "Tag 1"})
            n63 = call "KH TURCK ETHERNETIP RFID UserCommand Array.vi"("BitArray"="Read", "UserCommand"=KH_TURCK_ETHERNETIP_TDef_Enum_RFID_User_Command."read", "TagNr"=w139) -> ("initialized array"=w136:bool[])  [unwired: 7 in, 1 out]
            n64 = local write "Read"(w136) -> ()
          }
          event "Write": Value Change {
            n65 = event-data() -> ()  [unwired: 1 in, 1 out]
            n66 = flat-sequence {
              tunnel: w146 -> [w149]
              tunnel: [w150] -> w144
              tunnel: ["TagNr"] -> w143
              tunnel: [w148] -> w142
              tunnel: [w173] -> w145
              tunnel: w144 -> [w173]
              tunnel: w143 -> [w172]
              tunnel: w142 -> [w171]
              frame #0 {
                n67 = call "KH TURCK ETHERNETIP RFID UserCommand Array.vi"("BitArray"="Write", "UserCommand"=KH_TURCK_ETHERNETIP_TDef_Enum_RFID_User_Command."write", "TagNr"="TagNr") -> ("index of element"=w148:i32, "initialized array"=w152:bool[])  [unwired: 7 in]
                n68 = local write "Write"(w152) -> ()
                n69 = case shown="\"Tag 1\"" "TagNr" {
                  tunnel: w148 -> [w160 w168]
                  tunnel: [w157 w167] -> w150
                  tunnel: w149 -> [w156 w166]
                  tunnel: w148 -> [w155 w163]
                  frame "Tag 0", Default {
                    n70 = case shown="0" w160 {
                      tunnel: ["Write Kanal 0 Modul 2" "Write Kanal 0 Modul 1"] -> w159
                      frame 1, Default {
                        # "Modul 2"
                      }
                      frame 0 {
                        # "Modul 1"
                      }
                    }
                    n71 = call "KH TURCK ETHERNETIP FGlob RFID TAG0 AO.vi"("Nr Module"=w155, "Function"=KH_TURCK_TypeDefs_FGlob."Put one", "err in"=w156, "RFID one in"=w159) -> ("err out"=w157:errorcluster)  [unwired: 5 in, 2 out]
                  }
                  frame "Tag 1" {
                    n72 = case shown="1, Default" w168 {
                      tunnel: ["Write Kanal 1 Modul 2" "Write Kanal 1 Modul 1"] -> w164
                      frame 1, Default {
                        # "Modul 2"
                      }
                      frame 0 {
                        # "Modul 1"
                      }
                    }
                    n73 = call "KH TURCK ETHERNETIP FGlob RFID TAG1 AO.vi"("Nr Module"=w163, "Function"=KH_TURCK_TypeDefs_FGlob."Put one", "err in"=w166, "RFID one in"=w164) -> ("err out"=w167:errorcluster)  [unwired: 5 in, 2 out]
                  }
                }
              }
              frame #1 {
                n74 = call "KH TURCK ETHERNETIP RFID WriteTag.vi"("Modul Nr"=w171, "TagNr"=w172) -> ()  [unwired: 10 in]
              }
            }
          }
          event "Inventory": Value Change {
            n75 = event-data() -> ()  [unwired: 1 in, 1 out]
            n76 = local read "TagNr"() -> (w177:enum16{"Tag 0", "Tag 1"})
            n77 = call "KH TURCK ETHERNETIP RFID UserCommand Array.vi"("BitArray"="Inventory", "UserCommand"=KH_TURCK_ETHERNETIP_TDef_Enum_RFID_User_Command."inventory", "TagNr"=w177) -> ("initialized array"=w174:bool[])  [unwired: 7 in, 1 out]
            n78 = local write "Inventory"(w174) -> ()
          }
          event "Reset message": Value Change {
            n79 = event-data() -> ()  [unwired: 1 in, 1 out]
            n80 = global read "KH TURCK ETHERNETIP RFID Global.vi" "RFID 0 LS Array"() -> (w183:T18[])
            n81 = global read "KH TURCK ETHERNETIP RFID Global.vi" "RFID 1 LS Array"() -> (w181:T18[])
            n82 = for {
              tunnel: [w193] -> w184 mode=indexing
              tunnel: w183 -> [w192] mode=indexing
              tunnel: [w191] -> w182 mode=indexing
              tunnel: w181 -> [w190] mode=indexing
              tunnel: [FALSE ("TimeoutReading")] -> w180 mode=indexing
              w189 = FALSE ("TimeoutReading")
              n83 = Bundle By Name(cluster=w192, "Timeout"=w189, "WritingFinished"=w189, "ReadingFinished"=w189) -> (w193:T18)
              n84 = Bundle By Name(cluster=w190, "Timeout"=w189, "WritingFinished"=w189, "ReadingFinished"=w189) -> (w191:T18)
            }
            n85 = global write "KH TURCK ETHERNETIP RFID Global.vi" "RFID 1 LS Array"(w182) -> ()
            n86 = global write "KH TURCK ETHERNETIP RFID Global.vi" "RFID 0 LS Array"(w184) -> ()
            n87 = global write "KH TURCK ETHERNETIP RFID Global.vi" "WritingSuccessfull0"(w180) -> ()
            n88 = global write "KH TURCK ETHERNETIP RFID Global.vi" "ErrorWriting0"(w180) -> ()
            n89 = global write "KH TURCK ETHERNETIP RFID Global.vi" "WritingSuccessfull1"(w180) -> ()
            n90 = global write "KH TURCK ETHERNETIP RFID Global.vi" "ErrorWriting1"(w180) -> ()
            n91 = local write "Reset message"(FALSE ("TimeoutWriting")) -> ()
          }
        }
      }
      n92 = call "KH EthernetIP SetData.vi"("Function"="End", "error in"=w28) -> ("error out"=w32:errorcluster)  [unwired: 7 in, 2 out]
      n93 = call "KH EthernetIP GetData.vi"("Function"="End", "error in"=w35) -> ("error out"=w30:errorcluster)  [unwired: 8 in, 1 out]
      n94 = Merge Errors(w23, w32, w30, w26) -> (w31:errorcluster)
      n95 = call "KH EthernetIP OpenCloseConnection.vi"("Function"="Post", "error in"=w31) -> ("error out"=w25:errorcluster)  [unwired: 9 in]
    }
    frame Error {
      n96 = call <vilib>:"Simple Error Handler.vi"("error in (no error)"=w195) -> ("error out"=w194:errorcluster)  [unwired: 4 in, 4 out]
    }
  }
  n97 = flat-sequence {
    tunnel: w4 -> [w196]
    frame #0 {
      n98 = local write "Exit"(FALSE ("Exit")) -> ()
      "error out" <- w196
    }
  }
